vi "SubVI.vi"(5 "target_y":dbl, 6 "Start_Angle":dbl, 7 "target_x":dbl, 8 "start_y":dbl, 9 "start_x":dbl, 10 "Velocity_Limit":dbl, 11 "dt":dbl) -> (2 "VL_Array":dbl[](array[numeric]), 3 "VR_Array":dbl[](array[numeric]))   [LabVIEW 2015]
uses:
  <vilib>/imath/engines/lvmath/Plug In/_Char/NIMS_CH_character datatype.ctl
  <vilib>/imath/engines/lvmath2/RunTimeEngine/NodeEndStatement/NIMS_NodeEndStatement_Output.vi
  <instcachedir>/0/NIMS_NodeEndStatement_Output_53EC0D466D134D7ABD903AC30B43404B.lvgen/NIMS_NodeEndStatement_Output_53EC0D466D134D7ABD903AC30B43404B_012.vi
  <vilib>/imath/engines/lvmath2/RunTimeEngine/ErrorHandling/NIMS_Finalize Error.vi
  <vilib>/imath/engines/lvmath2/RunTimeEngine/Managers/WorkSpace/UID Generator.vi
  <vilib>/imath/engines/lvmath/Plug In/_Char/NIMS_CH_Character RV to String.vi
  <vilib>/imath/engines/lvmath2/RunTimeEngine/BuiltInFunctions/global/NIMS_global.vi
  <vilib>/imath/engines/lvmath2/RunTimeEngine/RunTimeType/NIMS_RunTimeType_From StrictType (excl LVString).vi
  <instcachedir>/0/NIMS_RunTimeType_From StrictType (excl LVString)_EB1C38A9BC5048DA9ABDA8F781E54D21.lvgen/NIMS_RunTimeType_From StrictType (excl LVString)_EB1C38A9BC5048DA9ABDA8F781E54D21_000.vi
  <vilib>/imath/engines/lvmath2/RunTimeEngine/BuiltInFunctions/_global_write/NIMS_global_write.vi
  <vilib>/imath/engines/lvmath2/RunTimeEngine/CommandStatement/MC_CommandStatement_break.vi
  Documents/LabVIEW Data/MathScriptVIs/MCStatic_35241984432_d3d16b5de3395579a5a17b373d698649.vi
  <instcachedir>/0/MCStatic_35241984432_d3d16b5de3395579a5a17b373d698649_6CE721F84CC34196811F0DCE839E5C05.lvgen/MCStatic_35241984432_d3d16b5de3395579a5a17b373d698649_6CE721F84CC34196811F0DCE839E5C05_002.vi
  Documents/LabVIEW Data/MathScriptVIs/MCStatic_35241984432_ebc62d5d4a74bd746b4bcd2d791c21f0.vi
  <instcachedir>/0/MCStatic_35241984432_ebc62d5d4a74bd746b4bcd2d791c21f0_E756CD2AD2434431ACEE1709864A7D1E.lvgen/MCStatic_35241984432_ebc62d5d4a74bd746b4bcd2d791c21f0_E756CD2AD2434431ACEE1709864A7D1E_000.vi
  <vilib>/imath/engines/lvmath2/RunTimeEngine/BuiltInFunctions/_global_read/NIMS_global_read.vi
  <vilib>/imath/engines/lvmath/Plug In/_PlotObject/RunTimeType/NIMS_PO_RunTimeType_To Plot object 2D.vi
  <vilib>/imath/engines/lvmath/Plug In/_Char/RunTimeType/NIMS_CH_RunTimeType_To Character 2D.vi
  <vilib>/imath/engines/lvmath2/RunTimeEngine/RunTimeType/NIMS_RunTimeType_To Numeric.vi
  <instcachedir>/0/NIMS_RunTimeType_To Numeric_B134FEC7BFC54ED5998F4CFD2EE98288.lvgen/NIMS_RunTimeType_To Numeric_B134FEC7BFC54ED5998F4CFD2EE98288_001.vi
  <vilib>/imath/engines/lvmath2/RunTimeEngine/Struct/NIMS_DynamicStruct_ToUDFInput - Matrix.vi
  <instcachedir>/0/NIMS_RunTimeType_To Numeric_B134FEC7BFC54ED5998F4CFD2EE98288.lvgen/NIMS_RunTimeType_To Numeric_B134FEC7BFC54ED5998F4CFD2EE98288_000.vi
  <vilib>/imath/engines/lvmath2/RunTimeEngine/RunTimeType/NIMS_RunTimeType_Get Case Value.vi
  Documents/LabVIEW Data/MathScriptVIs/MCStatic_35241984432_bbf16b9652ce3d182242477e2f667caf.vi
  <instcachedir>/0/MCStatic_35241984432_bbf16b9652ce3d182242477e2f667caf_20285C451E9E44A88081C9052203472A.lvgen/MCStatic_35241984432_bbf16b9652ce3d182242477e2f667caf_20285C451E9E44A88081C9052203472A_000.vi
  <vilib>/imath/engines/lvmath2/RunTimeEngine/CommandStatement/NIMS_CommandStatement_MaskErr.vi
  <vilib>/imath/engines/lvmath2/RunTimeEngine/VariableToken/NIMS_VariableToken_CondDefined.vi
  <instcachedir>/0/NIMS_VariableToken_CondDefined_FE30D0A1BFB24F098D41DEBABFE96BE1.lvgen/NIMS_VariableToken_CondDefined_FE30D0A1BFB24F098D41DEBABFE96BE1_002.vi
  <vilib>/imathl/engines/lvmath/Functions/Error Handling/Create Error.vi
  <vilib>/imath/engines/lvmath2/RunTimeEngine/ArithmeticOperatorToken/NIMS_ArithmeticOperator_multmx.vi
  <instcachedir>/0/NIMS_ArithmeticOperator_multmx_E413577642394AA3A74EB19F669417B0.lvgen/NIMS_ArithmeticOperator_multmx_E413577642394AA3A74EB19F669417B0_003.vi
  <vilib>/imath/engines/lvmath/Plug In/_Char/NIMS_CH_Character 2D to U8 2D.vi
  <instcachedir>/0/NIMS_ArithmeticOperator_multmx_E413577642394AA3A74EB19F669417B0.lvgen/NIMS_ArithmeticOperator_multmx_E413577642394AA3A74EB19F669417B0_002.vi
  <vilib>/imath/engines/lvmath2/RunTimeEngine/IndexRead/NIMS M(S,$).vi
  <instcachedir>/0/NIMS M(S,$)_F24F360562DE41D8BE234322A2E15C65.lvgen/NIMS M(S,$)_F24F360562DE41D8BE234322A2E15C65_001.vi
  <vilib>/imath/engines/lvmath2/RunTimeEngine/MatrixToken/NIMS_MatrixToken_RV_RV.vi
  <instcachedir>/0/NIMS_MatrixToken_RV_RV_D6DC5F1C7C3E461A9AC3F398A1D68386.lvgen/NIMS_MatrixToken_RV_RV_D6DC5F1C7C3E461A9AC3F398A1D68386_000.vi
  <vilib>/imath/engines/lvmath2/RunTimeEngine/ErrorHandling/NIMS_Create Error From Enums.vi
  <vilib>/imath/engines/lvmath2/RunTimeEngine/IndexRead/NIMS V(S).vi
  <instcachedir>/0/NIMS V(S)_0488751826AF41519A22953C041130DC.lvgen/NIMS V(S)_0488751826AF41519A22953C041130DC_002.vi
  <vilib>/imath/engines/lvmath2/RunTimeEngine/IndexReplace/NIMS M(S,$)=V.vi
  <instcachedir>/0/NIMS M(S,$)=V_260679A9E30142119AFD27BBD2C5FD93.lvgen/NIMS M(S,$)=V_260679A9E30142119AFD27BBD2C5FD93_001.vi
  <vilib>/imath/engines/lvmath2/RunTimeEngine/BuiltInFunctions/size/NIMS_I32=size(GM,I32).vi
  <instcachedir>/0/NIMS_I32=size(GM,I32)_9AD83C4E72C04920AD6CE84F01B75FA9.lvgen/NIMS_I32=size(GM,I32)_9AD83C4E72C04920AD6CE84F01B75FA9_003.vi
  <vilib>/imath/engines/lvmath2/RunTimeEngine/BuiltInFunctions/zeros/NIMS_V=zeros(I32,I32).vi
  <vilib>/imath/engines/lvmath2/RunTimeEngine/RangeToken/NIMS_Range_R2 - Integer.vi
  <instcachedir>/0/NIMS_Range_R2 - Integer_396D5D4FB869421F9245109A0975AD54.lvgen/NIMS_Range_R2 - Integer_396D5D4FB869421F9245109A0975AD54_000.vi
  <vilib>/imath/engines/lvmath2/RunTimeEngine/IndexRead/NIMS M(S,S).vi
  <instcachedir>/0/NIMS M(S,S)_AC51E74150A542F7991B9634C66F3096.lvgen/NIMS M(S,S)_AC51E74150A542F7991B9634C66F3096_001.vi
  <vilib>/imath/engines/lvmath2/RunTimeEngine/BuiltInFunctions/atan2/NIMS_atan2.vi
  <instcachedir>/0/NIMS_atan2_A91AA4A7D42247EDBE8F76DB99AF04A4.lvgen/NIMS_atan2_A91AA4A7D42247EDBE8F76DB99AF04A4_001.vi
  Documents/LabVIEW Data/MathScriptVIs/MCStatic_35241984432_50686de29dbf96c3495a1a6f2244338c.vi
  <instcachedir>/0/MCStatic_35241984432_50686de29dbf96c3495a1a6f2244338c_62984529F31D4815AD74F8278AA6EB01.lvgen/MCStatic_35241984432_50686de29dbf96c3495a1a6f2244338c_62984529F31D4815AD74F8278AA6EB01_000.vi
  <vilib>/imath/engines/lvmath2/RunTimeEngine/IndexReplace/NIMS V(S)=S.vi
  <instcachedir>/0/NIMS V(S)=S_9916D32195284AEB9D40BA9A64F3B0C5.lvgen/NIMS V(S)=S_9916D32195284AEB9D40BA9A64F3B0C5_000.vi
  <instcachedir>/0/NIMS V(S)_0488751826AF41519A22953C041130DC.lvgen/NIMS V(S)_0488751826AF41519A22953C041130DC_000.vi
  <instcachedir>/0/MCStatic_35241984432_50686de29dbf96c3495a1a6f2244338c_62984529F31D4815AD74F8278AA6EB01.lvgen/MCStatic_35241984432_50686de29dbf96c3495a1a6f2244338c_62984529F31D4815AD74F8278AA6EB01_001.vi
  <vilib>/imath/engines/lvmath2/RunTimeEngine/RowToken/NIMS_RowToken_M_CV.vi
  <instcachedir>/0/NIMS_RowToken_M_CV_9B618B8CC92945CC817A6654DDA3890E.lvgen/NIMS_RowToken_M_CV_9B618B8CC92945CC817A6654DDA3890E_001.vi
  <vilib>/imath/engines/lvmath2/RunTimeEngine/IndexReplace/NIMS M(S,S)=S.vi
  <instcachedir>/0/NIMS M(S,S)=S_72298AC072A24B679F5E0C14DB2DD503.lvgen/NIMS M(S,S)=S_72298AC072A24B679F5E0C14DB2DD503_001.vi
  <vilib>/imath/engines/lvmath/Functions/Error Handling/MergeErrorsWrapper.vi
  <instcachedir>/0/NIMS V(S)_0488751826AF41519A22953C041130DC.lvgen/NIMS V(S)_0488751826AF41519A22953C041130DC_003.vi
  Documents/LabVIEW Data/MathScriptVIs/MCStatic_35241984432_d64b7831c0195e70684798c34942528c.vi
  <instcachedir>/0/MCStatic_35241984432_d64b7831c0195e70684798c34942528c_F7E0DA6E3BEA4558A6108008EF46F3AB.lvgen/MCStatic_35241984432_d64b7831c0195e70684798c34942528c_F7E0DA6E3BEA4558A6108008EF46F3AB_002.vi
  Documents/LabVIEW Data/MathScriptVIs/MCStatic_35241984432_14bc63b7539d9c406098ae4edfa0fea6.vi
  <instcachedir>/0/MCStatic_35241984432_14bc63b7539d9c406098ae4edfa0fea6_B199317CF54E4AA7A328DE202462E35D.lvgen/MCStatic_35241984432_14bc63b7539d9c406098ae4edfa0fea6_B199317CF54E4AA7A328DE202462E35D_000.vi
  Documents/LabVIEW Data/MathScriptVIs/MCStatic_35241984432_a2be1c9ccb546ba05c578c7aefec4d41.vi
  <instcachedir>/0/MCStatic_35241984432_a2be1c9ccb546ba05c578c7aefec4d41_7BA7F4AB9CCA4B4898DAD10C1B5D21BB.lvgen/MCStatic_35241984432_a2be1c9ccb546ba05c578c7aefec4d41_7BA7F4AB9CCA4B4898DAD10C1B5D21BB_000.vi
  Documents/LabVIEW Data/MathScriptVIs/MCStatic_35241984432_ccc6774e040567fe009593e044db3ae3.vi
  <instcachedir>/0/MCStatic_35241984432_ccc6774e040567fe009593e044db3ae3_E1FA46F418404BA0B769709549388B92.lvgen/MCStatic_35241984432_ccc6774e040567fe009593e044db3ae3_E1FA46F418404BA0B769709549388B92_000.vi
  <vilib>/imath/engines/lvmath2/RunTimeEngine/MatrixToken/NIMS_MatrixToken_M_SorCV.vi
  <instcachedir>/0/NIMS_MatrixToken_M_SorCV_3C830043BFCC411C9F6D9D7CB15DF896.lvgen/NIMS_MatrixToken_M_SorCV_3C830043BFCC411C9F6D9D7CB15DF896_000.vi
  <vilib>/imath/engines/lvmath2/RunTimeEngine/MatrixToken/NIMS_MatrixToken_M_RV.vi
  <instcachedir>/0/NIMS_MatrixToken_M_RV_B7BA3D7C046243F991E926789B324F64.lvgen/NIMS_MatrixToken_M_RV_B7BA3D7C046243F991E926789B324F64_001.vi
  <vilib>/imath/engines/lvmath2/RunTimeEngine/IndexRead/NIMS M($,S).vi
  <instcachedir>/0/NIMS M($,S)_3E5749BBB62E49528D4765A77F1F6D98.lvgen/NIMS M($,S)_3E5749BBB62E49528D4765A77F1F6D98_000.vi
  <vilib>/imath/engines/lvmath2/RunTimeEngine/Managers/SymbolTable/Clear UID.vi
  <instcachedir>/0/NIMS_NodeEndStatement_Output_53EC0D466D134D7ABD903AC30B43404B.lvgen/NIMS_NodeEndStatement_Output_53EC0D466D134D7ABD903AC30B43404B_005.vi
  Documents/LabVIEW Data/Angle_Convert.m
  Documents/LabVIEW Data/Astar.m
  Documents/LabVIEW Data/Astar_potential.m
  Documents/LabVIEW Data/distance.m
  Documents/LabVIEW Data/expand_array.m
  Documents/LabVIEW Data/insert_open.m
  Documents/LabVIEW Data/min_fn.m
  Documents/LabVIEW Data/node_index.m
  Documents/LabVIEW Data/CalInnerAngleOfTriangle.m
  Documents/LabVIEW Data/Cal_Speed.m
  Documents/LabVIEW Data/Boundary.m
  Documents/LabVIEW Data/Int_Position.m
  Documents/LabVIEW Data/same.m
  Documents/LabVIEW Data/simplify_route.m
  <vilib>/imath/engines/lvmath2/RunTimeEngine/Managers/SymbolTable/NIMS_WorkSpace.lvlib
panel:
  out "size(s)":i32
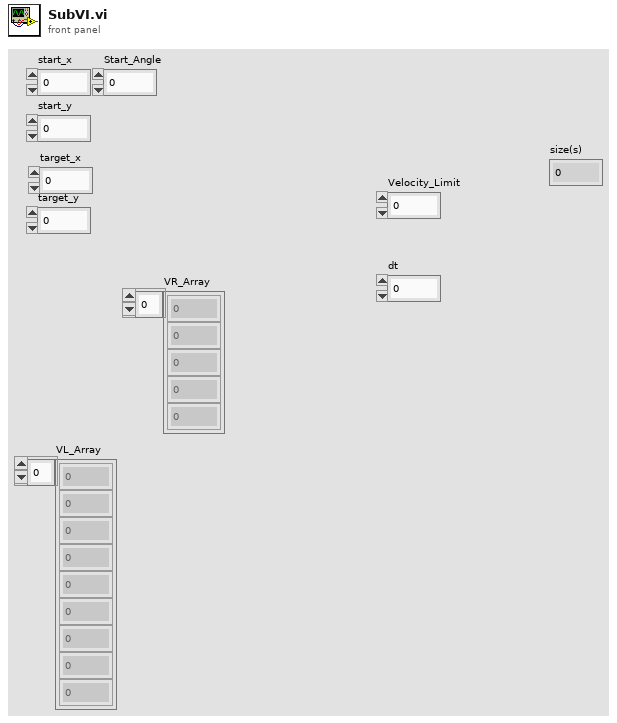
[diagram p1: front panel]
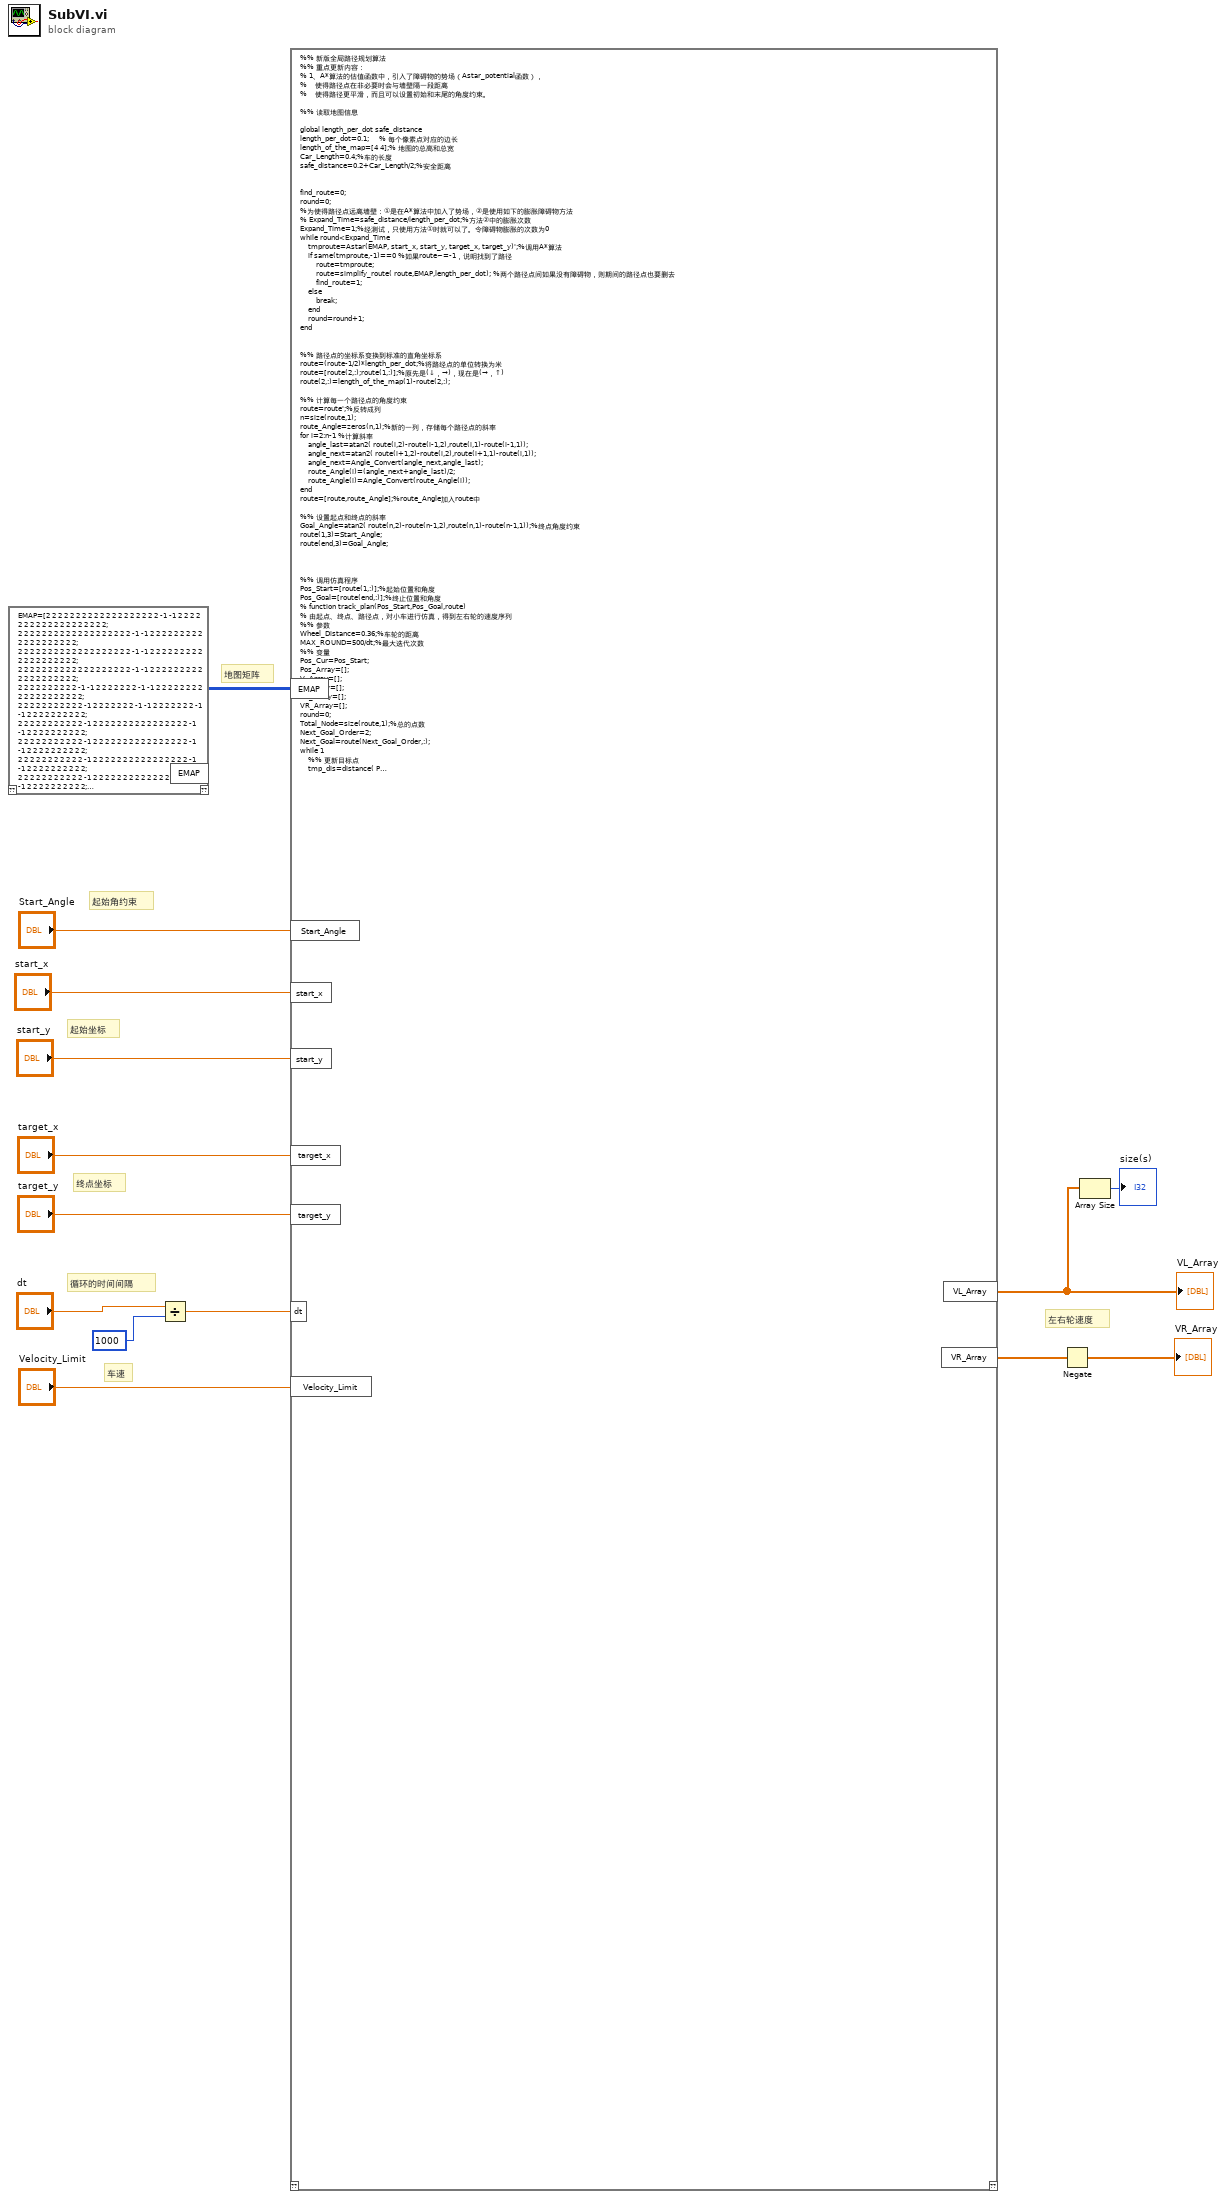
[diagram p0: block diagram]
diagram:
  # "其他关于小车的参数在此处改动"
  # "左右轮速度"
  # "地图矩阵"
  # "循环的时间间隔"
  # "车速"
  # "终点坐标"
  # "起始坐标"
  # "起始角约束"
  n1 = mathscript code="EMAP=[2\t2\t2\t2\t2\t2\t2\t2\t2\t2\t2\t2\t2\t2\t2\t2\t2\t2\t2\t-1\t-1\t2\t2\t2\t2\t2\t2\t2\t2\t2\t2\t2\t2\t2\t2\t2\t2\t2\t2\t2;\n2\t2\t2\t2\t2\t2\t2\t2\t2\t2\t2\t2\t2\t2\t2\t2\t2\t2\t2\t-1\t-1\t2\t2\t2\t2\t2\t2\t2\t2\t2\t2\t2\t2\t2\t2\t2\t2\t2\t2\t2;\n2\t2\t2\t2\t2\t2\t2\t2\t2\t2\t2\t2\t2\t2\t2\t2\t2\t2\t2\t-1\t-1\t2\t2\t2\t2\t2\t2\t2\t2\t2\t2\t2\t2\t2\t2\t2\t2\t2\t2\t2;\n2\t2\t2\t2\t2\t2\t2\t2\t2\t2\t2\t2\t2\t2\t2\t2\t2\t2\t2\t-1\t-1\t2\t2\t2\t2\t2\t2\t2\t2\t2\t2\t2\t2\t2\t2\t2\t2\t2\t2\t2;\n2\t2\t2\t2\t2\t2\t2\t2\t2\t2\t-1\t-1\t2\t2\t2\t2\t2\t2\t2\t-1\t-1\t2\t2\t2\t2\t2\t2\t2\t2\t2\t2\t2\t2\t2\t2\t2\t2\t2\t2\t2;\n2\t2\t2\t2\t2\t2\t2\t2\t2\t2\t2\t-1\t2\t2\t2\t2\t2\t2\t2\t-1\t-1\t2\t2\t2\t2\t2\t2\t2\t-1\t-1\t2\t2\t2\t2\t2\t2\t2\t2\t2\t2;\n2\t2\t2\t2\t2\t2\t2\t2\t2\t2\t2\t-1\t2\t2\t2\t2\t2\t2\t2\t2\t2\t2\t2\t2\t2\t2\t2\t2\t-1\t-1\t2\t2\t2\t2\t2\t2\t2\t2\t2\t2;\n2\t2\t2\t2\t2\t2\t2\t2\t2\t2\t2\t-1\t2\t2\t2\t2\t2\t2\t2\t2\t2\t2\t2\t2\t2\t2\t2\t2\t-1\t-1\t2\t2\t2\t2\t2\t2\t2\t2\t2\t2;\n2\t2\t2\t2\t2\t2\t2\t2\t2\t2\t2\t-1\t2\t2\t2\t2\t2\t2\t2\t2\t2\t2\t2\t2\t2\t2\t2\t2\t-1\t-1\t2\t2\t2\t2\t2\t2\t2\t2\t2\t2;\n2\t2\t2\t2\t2\t2\t2\t2\t2\t2\t2\t-1\t2\t2\t2\t2\t2\t2\t2\t2\t2\t2\t2\t2\t2\t2\t2\t2\t-1\t-1\t2\t2\t2\t2\t2\t2\t2\t2\t2\t2;\n2\t2\t2\t2\t2\t2\t2\t2\t2\t2\t-1\t-1\t-1\t2\t2\t2\t2\t2\t2\t2\t2\t2\t2\t2\t2\t2\t2\t2\t-1\t-1\t-1\t2\t2\t2\t2\t2\t2\t2\t2\t2;\n2\t2\t2\t-1\t-1\t-1\t-1\t-1\t-1\t-1\t-1\t-1\t-1\t-1\t-1\t-1\t-1\t-1\t-1\t-1\t-1\t-1\t-1\t-1\t-1\t-1\t-1\t-1\t-1\t-1\t-1\t-1\t-1\t-1\t2\t2\t2\t2\t2\t2;\n2\t2\t2\t-1\t-1\t-1\t-1\t-1\t-1\t-1\t-1\t-1\t-1\t-1\t-1\t-1\t-1\t-1\t-1\t-1\t-1\t-1\t-1\t-1\t-1\t-1\t-1\t-1\t-1\t-1\t-1\t-1\t-1\t-1\t2\t2\t2\t2\t2\t2;\n2\t2\t2\t-1\t-1\t-1\t-1\t-1\t-1\t-1\t-1\t-1\t-1\t-1\t-1\t-1\t-1\t-1\t-1\t-1\t-1\t-1\t-1\t-1\t-1\t-1\t-1\t-1\t-1\t-1\t-1\t-1\t-1\t-1\t2\t2\t2\t2\t2\t2;\n2\t2\t2\t-1\t-1\t2\t2\t2\t2\t2\t2\t2\t2\t2\t2\t2\t2\t2\t2\t2\t2\t2\t2\t2\t2\t2\t2\t2\t2\t2\t-1\t-1\t-1\t-1\t2\t2\t2\t2\t2\t2;\n2\t2\t2\t-1\t-1\t2\t2\t2\t2\t2\t2\t2\t2\t2\t2\t2\t2\t2\t2\t2\t2\t2\t2\t2\t2\t2\t2\t2\t2\t2\t-1\t-1\t-1\t-1\t2\t2\t2\t2\t2\t2;\n2\t2\t2\t-1\t-1\t2\t2\t2\t2\t2\t2\t2\t2\t2\t2\t2\t2\t2\t2\t2\t2\t2\t2\t2\t2\t2\t2\t2\t2\t2\t-1\t-1\t-1\t-1\t2\t2\t2\t2\t2\t2;\n2\t2\t2\t-1\t-1\t2\t2\t2\t2\t2\t2\t2\t2\t2\t2\t2\t2\t2\t2\t2\t2\t2\t2\t2\t2\t2\t2\t2\t2\t2\t-1\t-1\t-1\t-1\t2\t2\t2\t2\t2\t2;\n2\t2\t2\t-1\t-1\t2\t2\t2\t2\t2\t2\t2\t2\t2\t2\t2\t2\t2\t2\t2\t2\t2\t2\t2\t2\t2\t2\t2\t2\t2\t-1\t-1\t-1\t-1\t2\t2\t2\t2\t2\t2;\n2\t2\t2\t-1\t-1\t2\t2\t2\t2\t2\t2\t2\t2\t2\t2\t2\t2\t2\t2\t2\t2\t2\t2\t2\t2\t2\t2\t2\t2\t2\t-1\t-1\t-1\t-1\t2\t2\t2\t2\t2\t2;\n2\t2\t2\t-1\t-1\t2\t2\t2\t2\t2\t-1\t-1\t-1\t-1\t-1\t-1\t-1\t-1\t-1\t-1\t-1\t-1\t-1\t-1\t-1\t-1\t-1\t-1\t-1\t-1\t-1\t-1\t-1\t-1\t2\t2\t2\t2\t2\t2;\n2\t2\t2\t-1\t-1\t2\t2\t2\t2\t2\t-1\t-1\t-1\t-1\t-1\t-1\t-1\t-1\t-1\t-1\t-1\t-1\t-1\t-1\t-1\t-1\t-1\t-1\t-1\t-1\t-1\t-1\t-1\t-1\t2\t2\t2\t2\t2\t2;\n2\t2\t2\t-1\t-1\t2\t2\t2\t2\t2\t-1\t-1\t-1\t-1\t-1\t-1\t-1\t-1\t-1\t-1\t-1\t-1\t-1\t-1\t-1\t-1\t-1\t-1\t-1\t-1\t-1\t-1\t-1\t-1\t2\t2\t2\t2\t2\t2;\n2\t2\t2\t-1\t-1\t2\t2\t2\t2\t2\t-1\t-1\t-1\t-1\t-1\t-1\t-1\t-1\t-1\t-1\t-1\t-1\t-1\t-1\t-1\t-1\t-1\t-1\t-1\t-1\t-1\t-1\t-1\t-1\t2\t2\t2\t2\t2\t2;\n2\t2\t2\t-1\t-1\t2\t2\t2\t2\t2\t2\t2\t2\t2\t2\t2\t2\t2\t2\t2\t2\t2\t2\t2\t2\t2\t2\t2\t2\t2\t-1\t-1\t-1\t-1\t2\t2\t2\t2\t2\t2;\n2\t2\t2\t-1\t-1\t2\t2\t2\t2\t2\t2\t2\t2\t2\t2\t2\t2\t2\t2\t2\t2\t2\t2\t2\t2\t2\t2\t2\t2\t2\t-1\t-1\t-1\t-1\t2\t2\t2\t2\t2\t2;\n2\t2\t2\t-1\t-1\t2\t2\t2\t2\t2\t2\t2\t2\t2\t2\t2\t2\t2\t2\t2\t2\t2\t2\t2\t2\t2\t2\t2\t2\t2\t-1\t-1\t-1\t-1\t2\t2\t2\t2\t2\t2;\n2\t2\t2\t-1\t-1\t2\t2\t2\t2\t2\t2\t2\t2\t2\t2\t2\t2\t2\t2\t2\t2\t2\t2\t2\t2\t2\t2\t2\t2\t2\t-1\t-1\t-1\t-1\t2\t2\t2\t2\t2\t2;\n2\t2\t2\t-1\t-1\t2\t2\t2\t2\t2\t2\t2\t2\t2\t2\t2\t2\t2\t2\t2\t2\t2\t2\t2\t2\t2\t2\t2\t2\t2\t2\t2\t2\t2\t2\t2\t2\t2\t2\t2;\n2\t2\t2\t-1\t-1\t-1\t2\t2\t2\t2\t2\t2\t2\t2\t2\t2\t2\t2\t2\t2\t2\t2\t2\t2\t2\t2\t2\t2\t2\t2\t2\t2\t2\t2\t2\t2\t2\t2\t2\t2;\n2\t2\t2\t-1\t-1\t-1\t-1\t-1\t-1\t-1\t-1\t-1\t-1\t-1\t-1\t-1\t-1\t-1\t-1\t-1\t-1\t-1\t-1\t2\t2\t2\t2\t2\t2\t2\t2\t2\t2\t2\t2\t2\t2\t2\t2\t2;\n2\t2\t2\t-1\t-1\t-1\t-1\t-1\t-1\t-1\t-1\t-1\t-1\t-1\t-1\t-1\t-1\t-1\t-1\t-1\t-1\t-1\t-1\t2\t2\t2\t2\t2\t2\t2\t2\t2\t2\t2\t2 2\t2\t2\t2\t2;\n2\t2\t2\t2\t2\t2\t2\t2\t2\t2\t2\t2\t2\t-1\t-1\t-1\t2\t2\t2\t2\t2\t2\t2\t2\t2\t2\t2\t2\t2\t2\t2\t2\t2\t2\t2\t2\t2\t2\t2\t2;\n2\t2\t2\t2\t2\t2\t2\t2\t2\t2\t2\t2\t2\t-1\t-1\t-1\t2\t2\t2\t2\t2\t2\t2\t2\t2\t2\t2\t2\t2\t2\t2\t2\t2\t2\t2\t2\t2\t2\t2\t2;\n2\t2\t2\t2\t2\t2\t2\t2\t2\t2\t2\t2\t2\t-1\t-1\t-1\t2\t2\t2\t2\t2\t2\t2\t2\t2\t2\t2\t2\t2\t2\t2\t2\t2\t2\t2\t2\t2\t2\t2\t2;\n2\t2\t2\t2\t2\t2\t2\t2\t2\t2\t2\t2\t2\t-1\t-1\t-1\t2\t2\t2\t2\t2\t2\t2\t2\t2\t2\t2\t2\t2\t2\t2\t2\t2\t2\t2\t2\t2\t2\t2\t2;\n2\t2\t2\t2\t2\t2\t2\t2\t2\t2\t2\t2\t2\t-1\t-1\t-1\t2\t2\t2\t2\t2\t2\t2\t2\t2\t2\t2\t2\t2\t2\t2\t2\t2\t2\t2\t2\t2\t2\t2\t2;\n2\t2\t2\t2\t2\t2\t2\t2\t2\t2\t2\t2\t2\t2\t2\t2\t2\t2\t2\t2\t2\t2\t2\t2\t2\t2\t2\t2\t2\t2\t2\t2\t2\t2\t2\t2\t2\t2\t2\t2;\n2\t2\t2\t2\t2\t2\t2\t2\t2\t2\t2\t2\t2\t2\t2\t2\t2\t2\t2\t2\t2\t2\t2\t2\t2\t2\t2\t2\t2\t2\t2\t2\t2\t2\t2\t2\t2\t2\t2\t2;\n2\t2\t2\t2\t2\t2\t2\t2\t2\t2\t2\t2\t2\t2\t2\t2\t2\t2\t2\t2\t2\t2\t2\t2\t2\t2\t2\t2\t2\t2\t2\t2\t2\t2\t2\t2\t2\t2\t2\t2];"() -> ("EMAP"=w6:i32[][])  [unwired: 1 in, 1 out]
  n2 = Divide(x="dt", y=1000) -> (x/y=w4:dbl)
  n3 = mathscript code="%% 新版全局路径规划算法\n%% 重点更新内容：\n% 1、A*算法的估值函数中，引入了障碍物的势场（Astar_potential函数），\n%    使得路径点在非必要时会与墙壁隔一段距离\n%    使得路径更平滑，而且可以设置初始和末尾的角度约束。\n\n%% 读取地图信息\n\nglobal length_per_dot safe_distance\nlength_per_dot=0.1;     % 每个像素点对应的边长\nlength_of_the_map=[4 4];% 地图的总高和总宽\nCar_Length=0.4;%车的长度\nsafe_distance=0.2+Car_Length/2;%安全距离\n\n\nfind_route=0;\nround=0;\n%为使得路径点远离墙壁：①是在A*算法中加入了势场，②是使用如下的膨胀障碍物方法\n% Expand_Time=safe_distance/length_per_dot;%方法②中的膨胀次数\nExpand_Time=1;%经测试，只使用方法①时就可以了。令障碍物膨胀的次数为0\nwhile round<Expand_Time\n    tmproute=Astar(EMAP, start_x, start_y, target_x, target_y)';%调用A*算法\n    if same(tmproute,-1)==0 %如果route~=-1，说明找到了路径\n        route=tmproute;\n        route=simplify_route( route,EMAP,length_per_dot); %两个路径点间如果没有障碍物，则期间的路径点也要删去\n        find_route=1;\n    else\n        break;\n    end\n    round=round+1;\nend\n\n\n%% 路径点的坐标系变换到标准的直角坐标系\nroute=(route-1/2)*length_per_dot;%将路经点的单位转换为米\nroute=[route(2,:);route(1,:)];%原先是(↓，→)，现在是(→，↑)\nroute(2,:)=length_of_the_map(1)-route(2,:);\n\n%% 计算每一个路径点的角度约束\nroute=route';%反转成列\nn=size(route,1);\nroute_Angle=zeros(n,1);%新的一列，存储每个路径点的斜率\nfor i=2:n-1 %计算斜率\n    angle_last=atan2( route(i,2)-route(i-1,2),route(i,1)-route(i-1,1));\n    angle_next=atan2( route(i+1,2)-route(i,2),route(i+1,1)-route(i,1));\n    angle_next=Angle_Convert(angle_next,angle_last);\n    route_Angle(i)=(angle_next+angle_last)/2;\n    route_Angle(i)=Angle_Convert(route_Angle(i));\nend\nroute=[route,route_Angle];%route_Angle加入route中\n\n%% 设置起点和终点的斜率\nGoal_Angle=atan2( route(n,2)-route(n-1,2),route(n,1)-route(n-1,1));%终点角度约束\nroute(1,3)=Start_Angle;\nroute(end,3)=Goal_Angle;\n\n\n\n%% 调用仿真程序\nPos_Start=[route(1,:)];%起始位置和角度\nPos_Goal=[route(end,:)];%终止位置和角度\n% function track_plan(Pos_Start,Pos_Goal,route)\n% 由起点、终点、路径点，对小车进行仿真，得到左右轮的速度序列\n%% 参数\nWheel_Distance=0.36;%车轮的距离\nMAX_ROUND=500/dt;%最大迭代次数\n%% 变量\nPos_Cur=Pos_Start;\nPos_Array=[];\nV_Array=[];\nW_Array=[];\nVL_Array=[];\nVR_Array=[];\nround=0;\nTotal_Node=size(route,1);%总的点数\nNext_Goal_Order=2;\nNext_Goal=route(Next_Goal_Order,:);\nwhile 1\n    %% 更新目标点\n    tmp_dis=distance( Pos_Cur(1), Pos_Cur(2),Next_Goal(1),Next_Goal(2));\n    if Next_Goal_Order<=n-1\n        tmp_angle=CalInnerAngleOfTriangle(Pos_Cur,Next_Goal,...\n            route(Next_Goal_Order+1,:));\n    else\n        tmp_angle=0;\n    end\n    % 当dis小于一个很小的值时，一定使得目标点发生更新\n    % 当dis小于一个较小的值时，如果当前点与目标点、与下下个目标点\n    %   所组成的角度较大时，也使得目标点发生更新\n    if tmp_dis<0.03 || (tmp_dis<0.3 && tmp_angle>60/180*pi)\n        if Next_Goal_Order<Total_Node\n            Next_Goal_Order=Next_Goal_Order+1;\n            Next_Goal=route(Next_Goal_Order,:);\n        end\n    end\n    %% 到达终点的判定（即循环结束的条件）\n    if distance( Pos_Cur(1), Pos_Cur(2),Pos_Goal(1),Pos_Goal(2))<0.05\n        break;\n    end\n    round=round+1;\n    if round>MAX_ROUND\n        break;\n    end\n    %% 计算新的速度和位置\n    Steering_Limits=0.8;\n    krho=3; %线速度\n    kalpha=12; %向目标点的转速\n    kbeta=5; %角度约束的逼近程度\n    if Next_Goal_Order==n %最后一个点时，速度减慢，角度约束的逼近更快\n        kalpha=10; %向目标点的转速\n         kbeta=8; %角度约束的逼近程度\n    end\n    [V_Left,V_Right,v,w] = Cal_Speed( Pos_Cur,Next_Goal,Wheel_Distance,...\n            Velocity_Limit,Steering_Limits,krho,kalpha,kbeta);\n    Pos_Cur=Int_Position( Pos_Cur,v,w,dt);\n    %% 存储位置和速度\n    V_Array=[V_Array;real(v)];\n    W_Array=[W_Array;real(w)];\n    VL_Array=[VL_Array;real(V_Left)];\n    VR_Array=[VR_Array;real(V_Right)];\n    Pos_Array=[Pos_Array;real(Pos_Cur)];\nend\nVL_Array=VL_Array(:,1);\nVR_Array=VR_Array(:,1);"("dt"=w4, "Velocity_Limit"="Velocity_Limit", "start_x"="start_x", "start_y"="start_y", "target_x"="target_x", "target_y"="target_y", "Start_Angle"="Start_Angle", "EMAP"=w6) -> ("VL_Array"=w2:dbl[], "VR_Array"=w14:dbl[])  [unwired: 1 in, 1 out]
  "VL_Array" <- w2
  n4 = Negate(x=w14) -> (-x=→"VR_Array":dbl[])
  n5 = Array Size(array=w2) -> (size(s)=→"size(s)":i32)
